vi "UHR-Fleezers Control (host) - 12.0_test_fpga_connection.vi"() -> ()   [LabVIEW 2014] (continued)
    }
    n2827 = feedback-in #12(w3586) -> ()
    n2828 = feedback-in #13(w3587) -> ()
    n2829 = Square Root(x=w3683) -> (sqrt(x)=w3682:dbl)
    n2830 = Or(x=w3868, y=w3864) -> (x .or. y?=w3865:bool)
    n2831 = Equal?(x="Tab Control 6", y=T41."High Res Display") -> (x = y?=w3800:bool)
    n2832 = Multiply(x="APD Disp. Scale", y=w3762) -> (x*y=w3771:waveform(dbl)[])
    n2833 = Multiply(x=10.0, y=w3682) -> (x*y=→"Trap 1 Position RMS (A)":dbl)
    n2834 = Multiply(x="APD Disp. Downsample", y=w3769) -> (x*y=w3767:dbl)
    n2835 = Divide(x=w3771, y=w3767) -> (x/y=w3741:waveform(dbl)[])
    n2836 = case "For displaying the high resolution display (no downsampling)" shown="True" w3800 {
      tunnel: w3766 -> [_ w4168]
      frame False {
      }
      frame True {
        n2837 = Index Array(array=w4168, index="High Res. Display") -> (element=w4169:waveform(dbl))
        n2838 = call <vilib>:"Std Deviation and Variance.vi"("X"=w4169) -> ("mean"=w4176:dbl, "standard deviation"=w4181:dbl)  [unwired: 1 in, 1 out]
        "Mean Intensity" <- w4176
        "Sigma" <- w4181
        n2839 = Subtract(x=w4169, y=w4176) -> (x-y=w4175:waveform(dbl))
        n2840 = Select(t=w4175, s="Subtract mean", f=w4169) -> (s? t:f=→"1 Channel":waveform(dbl))
        n2841 = Divide(x=w4181, y=w4176) -> (x/y=→"Sigma/Mean":dbl)
        n2842 = feedback #15(1) -> (w4170:i32)
        n2843 = Greater Or Equal?(x=w4170, y="Slow mean N ave.") -> (x >= y?=w4183:bool)
        n2844 = Increment(x=w4170) -> (x+1=w4185:i32)
        n2845 = Select(t=1, s=w4183, f=w4185) -> (s? t:f=w4172:i32)
        n2846 = feedback-in #15(w4172) -> ()
        n2847 = feedback #16() -> (w4173:waveform(dbl))  [unwired: 1 out]
        n2848 = case shown="Default" w4170 {
          tunnel: [w4188 w4191] -> w4174
          tunnel: w4173 -> [w4190 _]
          tunnel: w4169 -> [w4189 w4191]
          frame Default {
            n2849 = call-poly <vilib>:"Append Waveforms.vi"("waveform B"=w4189, "waveform A"=w4190) -> ("waveform out"=w4188:waveform(dbl))  [unwired: 1 in, 8 out]
          }
          frame 1 {
          }
        }
        n2850 = feedback-in #16(w4174) -> ()
        n2851 = case shown="True" w4183 {
          tunnel: w4174 -> [_ w4187]
          frame False {
          }
          frame True {
            n2852 = call-poly <vilib>:"Mean.vi"("X"=w4187) -> ("mean"=→"Slow mean":dbl)  [unwired: 1 out]
          }
        }
      }
    }
    n2853 = Index Array(array=w3741, index=0) -> (element=w3750:waveform(dbl))
    n2854 = Index Array(array=w3741, index=1) -> (element=w3748:waveform(dbl))
    n2855 = case "For computing FFTs for display" shown="True" "Compute FFT" {
      tunnel: w3766 -> [_ w4882]
      frame False {
      }
      frame True {
        n2856 = Build Array("FFT 1 Choice 1", "FFT 1 Choice 2", "FFT 2 Choice 1", "FFT 2 Choice 2") -> (w4875:u16[])
        n2857 = Array Size(array=w4882) -> (size(s)=w4881:i32)
        n2858 = feedback-in #17(w4875) -> ()
        n2859 = feedback #17(u16[] [100, 100, 100, 100]) -> (w4876:u16[])
        n2860 = feedback-in #18("# Spectra to Ave.") -> ()
        n2861 = feedback #18("# Spectra to Ave.") -> (w4873:dbl)
        n2862 = Not Equal?(x="# Spectra to Ave.", y=w4873) -> (x != y?=w4872:bool)
        n2863 = Not Equal?(x=w4875, y=w4876) -> (x != y?=w4874:bool)
        n2864 = feedback #19(1.0) -> (w4859:dbl)
        n2865 = Compound Arithmetic op=OR("Reset FFT", w4874, w4872) -> (w4857:bool)
        n2866 = Select(t=1.0, s=w4857, f=w4859) -> (s? t:f=w4861:dbl)
        n2867 = Greater?(x=w4861, y="# Spectra to Ave.") -> (0:w4880:bool)
        n2868 = Increment(x=w4861) -> (x+1=w4860:dbl)
        n2869 = feedback-in #19(w4860) -> ()
        n2870 = local read "DMA Update Period (s)"() -> (w4855:dbl)
        n2871 = Multiply(x="# Spectra to Ave.", y=w4855) -> (x*y=→"Ave. Time (s)":dbl)
        n2872 = Build Array(cluster{"f0":dbl, "df":dbl, "magnitude":dbl[]} {"f0"=0.0, "df"=0.0, "magnitude"=[]} ("PSD")) -> (w4864:cluster{"f0":dbl, "df":dbl, "magnitude":dbl[]}[])
        n2873 = Build Array(w4864, w4864, w4864, w4864) -> (w4866:T52)
        n2874 = feedback #20(w4866) -> (w4871:T52)
        n2875 = for {
          N: 4 -> [_]
          tunnel: w4875 -> [w4904] mode=indexing
          tunnel: w4882 -> [w4905]
          tunnel: w4881 -> [w4907]
          tunnel: w4857 -> [w4900]
          tunnel: w4880 -> [w4899]
          tunnel: "# Spectra to Ave." -> [w4898]
          tunnel: [w4897] -> w4870 mode=indexing
          tunnel: w4871 -> [w4902] mode=indexing
          tunnel: [w4901] -> w4858 mode=indexing
          tunnel: w4861 -> [w4896]
          n2876 = Less?(x=w4904, y=w4907) -> (x < y?=w4906:bool)
          n2877 = Index Array(array=w4905, index=w4904) -> (element=w4903:waveform(dbl))
          n2878 = case shown="True" w4906 {
            tunnel: w4903 -> [_ w4924]
            tunnel: w4902 -> [w4909 w4922]
            tunnel: [w4909 w4910] -> w4901
            tunnel: w4900 -> [_ w4921]
            tunnel: w4899 -> [_ w4914]
            tunnel: w4898 -> [_ w4913]
            tunnel: [cluster{"f0":dbl, "df":dbl, "magnitude":dbl[]} {"f0"=0.0, "df"=0.0, "magnitude"=[]} ("PSD") w4915] -> w4897
            tunnel: w4896 -> [_ w4912]
            frame False {
            }
            frame True {
              n2879 = call <vilib>:"Std Deviation and Variance.vi"("X"=w4924) -> ("mean"=w4925:dbl)  [unwired: 1 in, 2 out]
              n2880 = Subtract(x=w4924, y=w4925) -> (x-y=w4923:waveform(dbl))
              n2881 = xnode "Spectral Measurements"("Signals"=w4923) -> ("PSD"=w4917:cluster{"f0":dbl, "df":dbl, "magnitude":dbl[]})  [unwired: 1 in, 1 out]
              n2882 = case shown="False" w4921 {
                tunnel: w4922 -> [w4934 _]
                tunnel: [w4930 w4939] -> w4910
                tunnel: w4917 -> [w4933 w4940]
                tunnel: w4914 -> [w4932 _]
                frame False {
                  n2883 = Build Array (concatenate)(w4934, w4933) -> (w4931:cluster{"f0":dbl, "df":dbl, "magnitude":dbl[]}[])
                  n2884 = case shown="True" w4932 {
                    tunnel: w4931 -> [w4935 w4938]
                    tunnel: [w4935 w4936] -> w4930
                    frame False {
                    }
                    frame True {
                      n2885 = Delete From Array(array=w4938, index=0) -> (array with subset deleted=w4936:cluster{"f0":dbl, "df":dbl, "magnitude":dbl[]}[])  [unwired: 1 in, 1 out]
                    }
                  }
                }
                frame True {
                  n2886 = Build Array(w4940) -> (w4939:cluster{"f0":dbl, "df":dbl, "magnitude":dbl[]}[])
                }
              }
              n2887 = for {
                tunnel: w4910 -> [w4929] mode=indexing
                tunnel: [w4928] -> w4920 mode=indexing
                workers-P: _ -> [_]
                n2888 = Unbundle By Name(w4929) -> ("magnitude"=w4928:dbl[])
              }
              n2889 = Transpose 2D Array(2D array=w4920) -> (transposed array=w4919:dbl[][])
              n2890 = for {
                tunnel: w4919 -> [w4927] mode=indexing
                tunnel: [w4926] -> w4918 mode=indexing
                workers-P: _ -> [_]
                n2891 = Add Array Elements(numeric array=w4927) -> (sum=w4926:dbl)
              }
              n2892 = Select(t=w4913, s=w4914, f=w4912) -> (s? t:f=w4911:dbl)
              n2893 = Divide(x=w4918, y=w4911) -> (x/y=w4916:dbl[])
              n2894 = Bundle By Name(cluster=w4917, "magnitude"=w4916) -> (w4915:cluster{"f0":dbl, "df":dbl, "magnitude":dbl[]})
            }
          }
        }
        n2895 = case shown="True" w4857 {
          tunnel: w4858 -> [w4889 w4895]
          tunnel: [w4889 w4890] -> w4856
          frame False {
          }
          frame True {
            n2896 = Array Subset(array=w4895, index (row)=0 ("index"), length (row)=4 ("length"), index (col)=0 ("index"), length (col)=1 ("length")) -> (w4890:T52)
          }
        }
        n2897 = feedback-in #20(w4856) -> ()
        n2898 = Split 1D Array(array=w4870, index=2) -> (first subarray=→"FFT 1":cluster{"f0":dbl, "df":dbl, "magnitude":dbl[]}[], second subarray=→"FFT 2":cluster{"f0":dbl, "df":dbl, "magnitude":dbl[]}[])
      }
    }
    n2899 = case "For plotting results of scanning MCL" shown="True" w3865 {
      tunnel: w3864 -> [_ w4310]
      tunnel: w3794 -> [_ w4406]
      tunnel: w3873 -> [_ _]
      tunnel: w3766 -> [_ w4380]
      tunnel: w3743 -> [_ w4311]
      tunnel: w3742 -> [_ w4284]
      frame False {
      }
      frame True {
        w4291 = u32 0 items=["Horizontal", "Vertical", "Central", "1st Diagonal", "2nd Diagonal"] ("Type of Symmetry")
        w4319 = u32 0 items=["Horizontal", "Vertical", "Central", "1st Diagonal", "2nd Diagonal"] ("Type of Symmetry")
        w4322 = u32 0 items=["Horizontal", "Vertical", "Central", "1st Diagonal", "2nd Diagonal"] ("Type of Symmetry")
        w4351 = u32 0 items=["Horizontal", "Vertical", "Central", "1st Diagonal", "2nd Diagonal"] ("Type of Symmetry")
        n2900 = Index Array(array=w4380, index=10) -> (element=w4386:waveform(dbl))
        n2901 = Index Array(array=w4380, index=11) -> (element=w4383:waveform(dbl))
        n2902 = local read "Cycles/step (MCL)"() -> (w4336:u64)
        n2903 = Index Array(array=w4380, index="Channel") -> (element=w4382:waveform(dbl))
        n2904 = Unbundle(w4284) -> ("New Image"=w4283:T2, "New Image"=w4282:T2, "New Image"=w4281:T2, "New Image"=w4280:T2)
        n2905 = Unbundle By Name(w4386) -> ("Y"=w4338:dbl[])
        n2906 = Unbundle By Name(w4383) -> ("Y"=w4340:dbl[])
        n2907 = Unbundle By Name(w4382) -> ("Y"=w4345:dbl[])
        n2908 = call "downsample 1D array - double.vi"("Ave N"=w4336, "Array In"=w4338) -> ("Array Out"=w4337:dbl[])  [unwired: 1 out]
        n2909 = call "downsample 1D array - double.vi"("Ave N"=w4336, "Array In"=w4340) -> ("Array Out"=w4339:dbl[])  [unwired: 1 out]
        n2910 = call "downsample 1D array - double.vi"("Ave N"=w4336, "Array In"=w4345) -> ("Array Out"=w4344:dbl[])  [unwired: 1 out]
        n2911 = feedback #21(w4406) -> (w4407:dbl[])
        n2912 = Build Array (concatenate)(w4407, w4406) -> (w4388:dbl[])
        n2913 = feedback #22(w4311) -> (w4313:dbl[])
        n2914 = Build Array (concatenate)(w4313, w4311) -> (w4312:dbl[])
        n2915 = local read "Scan steps (MCL)"() -> (w4293:u64)
        n2916 = Select(t=w4406, s=w4310, f=w4388) -> (s? t:f=w4392:dbl[])
        n2917 = feedback-in #21(w4392) -> ()
        n2918 = Select(t=w4311, s=w4310, f=w4312) -> (s? t:f=w4294:dbl[])
        n2919 = feedback-in #22(w4294) -> ()
        n2920 = local read "Scan lines (y)"() -> (w4279:u64)
        n2921 = local read "N APD Samp/step"() -> (w4295:dbl)
        n2922 = feedback #23(w4337) -> (w4394:dbl[])
        n2923 = Build Array (concatenate)(w4394, w4337) -> (w4385:dbl[])
        n2924 = feedback #24(w4344) -> (w4404:dbl[])
        n2925 = Build Array (concatenate)(w4404, w4344) -> (w4403:dbl[])
        n2926 = feedback #25(w4339) -> (w4396:dbl[])
        n2927 = Build Array (concatenate)(w4396, w4339) -> (w4397:dbl[])
        n2928 = Select(t=w4337, s=w4310, f=w4385) -> (s? t:f=w4341:dbl[])
        n2929 = feedback-in #23(w4341) -> ()
        n2930 = Select(t=w4344, s=w4310, f=w4403) -> (s? t:f=w4343:dbl[])
        n2931 = feedback-in #24(w4343) -> ()
        n2932 = Select(t=w4339, s=w4310, f=w4397) -> (s? t:f=w4342:dbl[])
        n2933 = feedback-in #25(w4342) -> ()
        n2934 = Multiply(x=w4293, y=u64 2) -> (x*y=w4278:u64)
        n2935 = call "integrate 1D array interval - double.vi"("Ave N"=w4295, "Array In"=w4294) -> ("Array Out"=w4306:dbl[])  [unwired: 1 out]
        n2936 = call "integrate 1D array interval - double.vi"("Ave N"=w4295, "Array In"=w4392) -> ("Array Out"=w4391:dbl[])  [unwired: 1 out]
        n2937 = Array Size(array=w4306) -> (size(s)=w4307:i32)
        n2938 = Array Size(array=w4391) -> (size(s)=w4393:i32)
        n2939 = Multiply(x=w4279, y=w4278) -> (x*y=w4309:u64)
        n2940 = Multiply(x=w4279, y=w4278) -> (x*y=w4401:u64)
        n2941 = call-poly <vilib>:"Mean.vi"("X"=w4341) -> ("mean"=w4325:dbl)  [unwired: 1 out]
        n2942 = Subtract(x=w4309, y=w4307) -> (x-y=w4300:u64)
        n2943 = call-poly <vilib>:"Mean.vi"("X"=w4343) -> ("mean"=w4330:dbl)  [unwired: 1 out]
        n2944 = call-poly <vilib>:"Mean.vi"("X"=w4342) -> ("mean"=w4328:dbl)  [unwired: 1 out]
        n2945 = call-poly <vilib>:"Mean.vi"("X"=w4306) -> ("mean"=w4297:dbl)  [unwired: 1 out]
        n2946 = Subtract(x=w4401, y=w4393) -> (x-y=w4335:u64)
        n2947 = call-poly <vilib>:"Mean.vi"("X"=w4391) -> ("mean"=w4332:dbl)  [unwired: 1 out]
        n2948 = Initialize Array(1.0 ("element"), w4300) -> (w4296:dbl[])
        n2949 = Initialize Array(1.0 ("element"), w4335) -> (w4326:dbl[])
        n2950 = Multiply(x=w4296, y=w4297) -> (x*y=w4298:dbl[])
        n2951 = Multiply(x=w4326, y=w4328) -> (x*y=w4329:dbl[])
        n2952 = Multiply(x=w4326, y=w4330) -> (x*y=w4331:dbl[])
        n2953 = Multiply(x=w4326, y=w4325) -> (x*y=w4327:dbl[])
        n2954 = Multiply(x=w4326, y=w4332) -> (x*y=w4333:dbl[])
        n2955 = Build Array (concatenate)(w4341, w4327) -> (w4395:dbl[])
        n2956 = Build Array (concatenate)(w4343, w4331) -> (w4399:dbl[])
        n2957 = Build Array (concatenate)(w4342, w4329) -> (w4398:dbl[])
        n2958 = Build Array (concatenate)(w4306, w4298) -> (w4308:dbl[])
        n2959 = Build Array (concatenate)(w4391, w4333) -> (w4400:dbl[])
        n2960 = Reshape Array(w4395, w4279, w4278) -> (w4361:dbl[][])
        n2961 = Reshape Array(w4308, w4279, w4278) -> (w4304:dbl[][])
        n2962 = Reshape Array(w4399, w4279, w4278) -> (w4353:dbl[][])
        n2963 = Reshape Array(w4398, w4279, w4278) -> (w4368:dbl[][])
        n2964 = Reshape Array(w4400, w4279, w4278) -> (w4378:dbl[][])
        n2965 = Array Subset(array=w4368, index (col)=0 ("index"), length (col)=w4293) -> (w4373:dbl[][])  [unwired: 2 in]
        n2966 = Array Subset(array=w4368, index (col)=w4293) -> (w4371:dbl[][])  [unwired: 3 in]
        n2967 = Array Subset(array=w4353, index (col)=0 ("index"), length (col)=w4293) -> (w4359:dbl[][])  [unwired: 2 in]
        n2968 = Array Subset(array=w4353, index (col)=w4293) -> (w4357:dbl[][])  [unwired: 3 in]
        n2969 = Array Subset(array=w4304, index (col)=0 ("index"), length (col)=w4293) -> (w4303:dbl[][])  [unwired: 2 in]
        n2970 = Array Subset(array=w4304, index (col)=w4293) -> (w4301:dbl[][])  [unwired: 3 in]
        n2971 = Array Subset(array=w4378, index (col)=0 ("index"), length (col)=w4293) -> (w4377:dbl[][])  [unwired: 2 in]
        n2972 = Array Subset(array=w4378, index (col)=w4293) -> (w4375:dbl[][])  [unwired: 3 in]
        n2973 = Array Subset(array=w4361, index (col)=0 ("index"), length (col)=w4293) -> (w4366:dbl[][])  [unwired: 2 in]
        n2974 = Array Subset(array=w4361, index (col)=w4293) -> (w4364:dbl[][])  [unwired: 3 in]
        n2975 = for {
          tunnel: w4373 -> [w4415] mode=indexing
          tunnel: [w4414] -> w4372 mode=indexing
          workers-P: _ -> [_]
          n2976 = Reverse 1D Array(array=w4415) -> (reversed array=w4414:dbl[])
        }
        n2977 = for {
          tunnel: w4359 -> [w4411] mode=indexing
          tunnel: [w4410] -> w4358 mode=indexing
          workers-P: _ -> [_]
          n2978 = Reverse 1D Array(array=w4411) -> (reversed array=w4410:dbl[])
        }
        n2979 = for {
          tunnel: w4303 -> [w4409] mode=indexing
          tunnel: [w4408] -> w4302 mode=indexing
          workers-P: _ -> [_]
          n2980 = Reverse 1D Array(array=w4409) -> (reversed array=w4408:dbl[])
        }
        n2981 = for {
          tunnel: w4377 -> [w4417] mode=indexing
          tunnel: [w4416] -> w4376 mode=indexing
          workers-P: _ -> [_]
          n2982 = Reverse 1D Array(array=w4417) -> (reversed array=w4416:dbl[])
        }
        n2983 = for {
          tunnel: w4366 -> [w4413] mode=indexing
          tunnel: [w4412] -> w4365 mode=indexing
          workers-P: _ -> [_]
          n2984 = Reverse 1D Array(array=w4413) -> (reversed array=w4412:dbl[])
        }
        n2985 = Index Array(array=w4378, index (row)=0) -> (element=→"Waveform Graph":dbl[])  [unwired: 1 in]
        n2986 = Add(x=w4372, y=w4371) -> (x+y=w4370:dbl[][])
        n2987 = Add(x=w4358, y=w4357) -> (x+y=w4356:dbl[][])
        n2988 = Add(x=w4302, y=w4301) -> (x+y=w4286:dbl[][])
        n2989 = Add(x=w4376, y=w4375) -> (x+y=w4350:dbl[][])
        n2990 = Add(x=w4365, y=w4364) -> (x+y=w4363:dbl[][])
        n2991 = Divide(x=w4356, y=2) -> (x/y=w4354:dbl[][])
        n2992 = Divide(x=w4370, y=2) -> (x/y=w4315:dbl[][])
        n2993 = Divide(x=w4363, y=2) -> (x/y=w4317:dbl[][])
        n2994 = To Single Precision Float(number=w4350) -> (single precision float=w4349:sgl[][])
        n2995 = Transpose 2D Array(2D array=w4354) -> (transposed array=→"Data map":dbl[][])
        n2996 = To Single Precision Float(number=w4286) -> (single precision float=w4290:sgl[][])
        n2997 = To Single Precision Float(number=w4315) -> (single precision float=w4321:sgl[][])
        n2998 = To Single Precision Float(number=w4317) -> (single precision float=w4318:sgl[][])
        n2999 = call "IMAQ ArrayToImage"("Image Pixels (Float)"=w4349, "Image"=w4283) -> ("Image Out"=w4352:T2)  [unwired: 8 in, 1 out]
        n3000 = call "IMAQ ArrayToImage"("Image Pixels (Float)"=w4290, "Image"=w4282) -> ("Image Out"=w4292:T2)  [unwired: 8 in, 1 out]
        n3001 = call "IMAQ ArrayToImage"("Image Pixels (Float)"=w4321, "Image"=w4281) -> ("Image Out"=w4323:T2)  [unwired: 8 in, 1 out]
        n3002 = call "IMAQ ArrayToImage"("Image Pixels (Float)"=w4318, "Image"=w4280) -> ("Image Out"=w4320:T2)  [unwired: 8 in, 1 out]
        n3003 = call "IMAQ Symmetry"("Type of Symmetry"=w4351, "Image Src"=w4352) -> ("Image Dst Out"=w4347:T2)  [unwired: 3 in, 1 out]
        n3004 = call "IMAQ Symmetry"("Type of Symmetry"=w4291, "Image Src"=w4292) -> ("Image Dst Out"=w4288:T2)  [unwired: 3 in, 1 out]
        n3005 = call "IMAQ Symmetry"("Type of Symmetry"=w4322, "Image Src"=w4323) -> ("Image Dst Out"=→"Detection Laser X":T2)  [unwired: 3 in, 1 out]
        n3006 = call "IMAQ Symmetry"("Type of Symmetry"=w4319, "Image Src"=w4320) -> ("Image Dst Out"=→"Detection Laser Y":T2)  [unwired: 3 in, 1 out]
        n3007 = call "IMAQ Set Simple Calibration"("Calibration Axis Info"=T42 {"Origin Pixel"={"X"=0.0, "Y"=0.0}, "Angle Relative to Horizontal (deg)"=0.0, "Axis Reference"=0}, "Grid Descriptor"=T43 {"X Step"=0.3, "Y Step"=0.3, "Unit"=enum."Undefined"}, "Image"=w4347) -> ("Calibrated Image"=→"APD 1":T2)  [unwired: 7 in, 1 out]
        n3008 = call "IMAQ Set Simple Calibration"("Calibration Axis Info"=T42 {"Origin Pixel"={"X"=0.0, "Y"=0.0}, "Angle Relative to Horizontal (deg)"=0.0, "Axis Reference"=0}, "Grid Descriptor"=T43 {"X Step"=0.3, "Y Step"=0.3, "Unit"=enum."Undefined"}, "Image"=w4288) -> ("Calibrated Image"=→"APD 2":T2)  [unwired: 7 in, 1 out]
      }
    }
    n3009 = Subtract(x=w3748, y="APD 2 Offset") -> (x-y=w3745:waveform(dbl))
    n3010 = Subtract(x=w3750, y="APD 1 Offset") -> (x-y=w3746:waveform(dbl))
    n3011 = Index Array(array=w3764, index=3) -> (element=w3818:waveform(dbl))
    n3012 = Index Array(array=w3764, index=6) -> (element=w3815:waveform(dbl))
    n3013 = Build Array(w3746, w3745) -> (→"APD Chart":waveform(dbl)[])
    n3014 = Array Size(array=w3586) -> (size(s)=w3854:i32)
    n3015 = call <vilib>:"Std Deviation and Variance.vi"("X"=w3587) -> ("standard deviation"=w3757:dbl)  [unwired: 1 in, 2 out]
    n3016 = Add Array Elements(numeric array=w3587) -> (sum=w3759:u32)
    n3017 = Add Array Elements(numeric array=w3586) -> (sum=w3863:u32)
    n3018 = call <vilib>:"Std Deviation and Variance.vi"("X"=w3586) -> ("standard deviation"=w3809:dbl)  [unwired: 1 in, 2 out]
    n3019 = Divide(x="T1 offset_x (mV)", y=1000.0) -> (x/y=w3819:dbl)
    n3020 = Divide(x=w3757, y=w3756) -> (x/y=w3753:dbl)
    "Rate sigma (Hz) 2" <- w3753
    n3021 = Multiply(x=w3756, y=w3854) -> (x*y=w3758:dbl)
    "Int. Time (s)" <- w3758
    n3022 = Divide(x=w3759, y=w3758) -> (x/y=w3754:dbl)
    "APD 2 Rate (Hz)" <- w3754
    n3023 = Divide(x=w3863, y=w3758) -> (x/y=w3807:dbl)
    "APD 1 Rate (Hz)" <- w3807
    n3024 = Divide(x=w3809, y=w3756) -> (x/y=w3808:dbl)
    "Rate sigma (Hz)" <- w3808
    n3025 = Divide(x=w3753, y=w3754) -> (x/y=→"Sigma/Mean 2":dbl)
    n3026 = Divide(x=w3808, y=w3807) -> (x/y=→"s/Mean":dbl)
    n3027 = feedback-in #26("Calibration") -> ()
    n3028 = feedback #26(u16 1 ("Calibration")) -> (w3837:u16)
    n3029 = Divide(x="T2 offset_x (mV)", y=1000.0) -> (x/y=w3817:dbl)
    n3030 = case shown="0, Default" "Calibration" {
      tunnel: "T1 a_x (nm/V)" -> [_ w4246 w4267]
      tunnel: "T1 k_x (pN/nm)" -> [_ _ w4257]
      tunnel: "T2 a_x (nm/V)" -> [_ w4245 w4265]
      tunnel: "T2 k_x (pN/nm)" -> [_ _ w4258]
      tunnel: w3818 -> [w4228 w4243 w4263]
      tunnel: w3815 -> [w4227 w4241 w4261]
      tunnel: [w4228 w4240 w4260] -> w3846
      tunnel: [w4227 w4239 w4259] -> w3845
      tunnel: ["T1 X (V)" ("Label.Text") "T1 X (nm)" ("Label.Text") "T1 X (pN)" ("Label.Text")] -> w3834
      tunnel: ["T2 X (V)" ("Label.Text") "T2 X (nm)" ("Label.Text") "T2 X (pN)" ("Label.Text")] -> w3833
      tunnel: ["Position (V)" ("Label.Text") "Position (nm)" ("Label.Text") "Force (pN)" ("Label.Text")] -> w3835
      tunnel: w3817 -> [_ w4231 w4250]
      tunnel: w3819 -> [_ w4234 w4252]
      tunnel: ["Mean (V)" ("Label.Text") "Mean (nm)" ("Label.Text") "Mean (pN)" ("Label.Text")] -> w3830
      tunnel: ["Difference (V)" ("Label.Text") "Difference (nm)" ("Label.Text") "Difference (pN)" ("Label.Text")] -> w3772
      frame 0, Default {
      }
      frame 1 {
        n3031 = Unbundle By Name(w4243) -> ("Y"=w4247:dbl[])
        n3032 = Unbundle By Name(w4241) -> ("Y"=w4232:dbl[])
        n3033 = Subtract(x=w4247, y=w4234) -> (x-y=w4235:dbl[])
        n3034 = Subtract(x=w4232, y=w4231) -> (x-y=w4233:dbl[])
        n3035 = Multiply(x=w4233, y=w4245) -> (x*y=w4242:dbl[])
        n3036 = Multiply(x=w4246, y=w4235) -> (x*y=w4244:dbl[])
        n3037 = Bundle By Name(cluster=w4241, "Y"=w4242) -> (w4239:waveform(dbl))
        n3038 = Bundle By Name(cluster=w4243, "Y"=w4244) -> (w4240:waveform(dbl))
      }
      frame 2 {
        n3039 = Unbundle By Name(w4263) -> ("Y"=w4268:dbl[])
        n3040 = Unbundle By Name(w4261) -> ("Y"=w4266:dbl[])
        n3041 = Subtract(x=w4266, y=w4250) -> (x-y=w4251:dbl[])
        n3042 = Subtract(x=w4268, y=w4252) -> (x-y=w4253:dbl[])
        n3043 = Compound Arithmetic op=MULTIPLY(w4251, w4265, w4258) -> (w4262:dbl[])
        n3044 = Compound Arithmetic op=MULTIPLY(w4257, w4267, w4253) -> (w4264:dbl[])
        n3045 = Bundle By Name(cluster=w4261, "Y"=w4262) -> (w4259:waveform(dbl))
        n3046 = Bundle By Name(cluster=w4263, "Y"=w4264) -> (w4260:waveform(dbl))
      }
    }
    n3047 = Not Equal?(x=w3837, y="Calibration") -> (x != y?=w3798:bool)
    n3048 = case shown="True" w3798 {
      tunnel: w3835 -> [_ w4221]
      tunnel: w3834 -> [_ w4220]
      tunnel: w3833 -> [_ w4219]
      tunnel: w3830 -> [_ w4218]
      tunnel: w3772 -> [_ w4217]
      frame False {
      }
      frame True {
        n3049 = property on="Force" class="WFChart (strict)"("YScale.NameLbl.Text"=w4221) -> ()  [unwired: 2 in, 2 out]
        n3050 = property on="T2 X" class="DigNum (strict)"("Caption.Text"=w4219) -> ()  [unwired: 2 in, 2 out]
        n3051 = property on="T1 X" class="DigNum (strict)"("Caption.Text"=w4220) -> ()  [unwired: 2 in, 2 out]
        n3052 = property on="Mean" class="DigNum (strict)"("Caption.Text"=w4218) -> ()  [unwired: 2 in, 2 out]
        n3053 = property on="Difference" class="DigNum (strict)"("Caption.Text"=w4217) -> ()  [unwired: 2 in, 2 out]
      }
    }
    n3054 = Unbundle By Name(w3818) -> ("Y"=w3821:dbl[])
    n3055 = Unbundle By Name(w3815) -> ("Y"=w3824:dbl[])
    n3056 = Subtract(x=w3821, y=w3819) -> (x-y=w3822:dbl[])
    n3057 = Subtract(x=w3824, y=w3817) -> (x-y=w3823:dbl[])
    n3058 = Multiply(x=w3823, y="T2 a_x (nm/V)") -> (x*y=w3625:dbl[])
    n3059 = Multiply(x="T1 a_x (nm/V)", y=w3822) -> (x*y=w3626:dbl[])
    n3060 = Not(x="Trap Trig. Fl.") -> (.not. x?=w3662:bool)
    n3061 = Multiply(x=w3845, y=-1.0) -> (x*y=w3826:waveform(dbl))
    n3062 = Subtract(x=w3626, y=w3625) -> (x-y=w3814:dbl[])
    n3063 = Unbundle By Name(w3845) -> ("Y"=w3788:dbl[])
    n3064 = Unbundle By Name(w3846) -> ("Y"=w3627:dbl[])
    n3065 = Negate(x=w3814) -> (-x=w3623:dbl[])
    n3066 = Build Array(w3846, w3826) -> (→"Force":waveform(dbl)[])
    n3067 = Subtract(x=w3623, y="Offset (nm)") -> (x-y=w3786:dbl[])
    n3068 = case shown="True" "Read Lateness and Rel Phase" {
      tunnel: w3643 -> [w4192 w4216]
      tunnel: w3642 -> [w4193 w4215]
      tunnel: [w4192 w4214] -> w3812
      tunnel: [w4193 w4213] -> w3811
      frame False {
      }
      frame True {
        n3069 = xnode "Read/Write Control"("FPGA VI Reference In"=w4216, "error in"=w4215) -> ("FPGA VI Reference Out"=w4214:T22, "error out"=w4213:errorcluster, "GI Relative phase"=→"GI relative phase":i16, "Relative phase"=→"Relative phase (AI1)":i16, "AI Late Counter"=→"Late Counter (AI1)":u8, "GI Late Counter"=→"GI Late Counter":u8, "MCL Late Counter"=→"MCL Late Counter":u8, "MCL Relative Phase"=→"Relative Phase (MCL)":i16, "APD Acq Relative Phase"=→"APD Acq Relative Phase":i16, "APD 1 Gate Relative Phase"=→"APD 1 Gate Relative Phase":i16, "APD 2 Gate Relative Phase"=→"APD 2 Gate Relative Phase":i16, "APD Acq Late Counter"=→"APD Acq Late Counter":u8, "APD 1 Gate Late Counter"=→"APD 1 Gate Late Counter":u8, "APD 2 Gate Late Counter"=→"APD 2 Gate Late Counter":u8, "Green FB Relative Phase"=→"Relative phase (Green FB)":i16, "GI Relative phase 2"=→"GI relative phase 2":i16, "GI Late Counter 2"=→"GI Late Counter 2":u8, "Trap Pos FIFO Timeout"=→"Trap Pos FIFO Timeout":u16, "Trap AI FIFO Timeout"=→"Trap AI FIFO Timeout":u16, "RI relative phase"=→"RI relative phase":i16, "RI late counter"=→"RI late counter":u8)
      }
    }
    n3070 = call-poly <vilib>:"Mean.vi"("X"=w3788) -> ("mean"=w3629:dbl)  [unwired: 1 out]
    "T2 X" <- w3629
    n3071 = Negate(x=w3788) -> (-x=w3789:dbl[])
    n3072 = call-poly <vilib>:"Mean.vi"("X"=w3627) -> ("mean"=w3630:dbl)  [unwired: 1 out]
    "T1 X" <- w3630
    n3073 = Negate(x=w3629) -> (-x=w3628:dbl)
    n3074 = Bundle By Name(cluster=w3818, "Y"=w3786) -> (w3763:waveform(dbl))
    "Bead Separation" <- w3763
    n3075 = Add(x=w3627, y=w3789) -> (x+y=w3790:dbl[])
    n3076 = Add(x=w3630, y=w3628) -> (x+y=w3832:dbl)
    n3077 = Subtract(x=w3630, y=w3628) -> (x-y=→"Difference":dbl)
    n3078 = Divide(x=w3790, y=2.0) -> (x/y=→"Vec Mean of T1 T2":dbl[])
    n3079 = Divide(x=w3832, y=2.0) -> (x/y=w3792:dbl)
    "Mean" <- w3792
    n3080 = feedback-in #27("Trap Trig. Fl.") -> ()
    n3081 = feedback #27("Trap Trig. Fl.") -> (w3660:bool)
    n3082 = And(x=w3662, y=w3660) -> (x .and. y?=w3661:bool)
    n3083 = case "If have just turned off triggering" shown="True" w3661 {
      tunnel: w3643 -> [_ w4022]
      tunnel: w3642 -> [_ w4021]
      frame False {
      }
      frame True {
        w4020 = FALSE ("FPGA Trap Trig")
        n3084 = xnode "Read/Write Control"("FPGA VI Reference In"=w4022, "error in"=w4021, "FPGA Trap Trig"=w4020) -> ("FPGA VI Reference Out"=w4019:T22, "error out"=w4018:errorcluster)
        n3085 = xnode "Read/Write Control"("FPGA VI Reference In"=w4019, "error in"=w4018, "TTrig?"=w4020) -> ()  [unwired: 2 out]
        n3086 = local write "Initializing"(FALSE ("Initializing")) -> ()
        n3087 = local write "Triggered"(FALSE ("Triggered")) -> ()
        n3088 = local write "Waiting"(FALSE ("Waiting")) -> ()
      }
    }
    n3089 = Not(x=w3660) -> (.not. x?=w3673:bool)
    n3090 = And(x="Trap Trig. Fl.", y=w3673) -> (x .and. y?=w3670:bool)
    n3091 = local read "Tether"() -> (w3793:bool)
    n3092 = Or(x=w3670, y="Reinitialize") -> (x .or. y?=w3656:bool)
    n3093 = feedback #28(w3666) -> (w3671:string)
    n3094 = Select(t=w3666, s=w3670, f=w3671) -> (s? t:f=w3665:string)
    n3095 = Select(t=w3666, s="Reinitialize", f=w3665) -> (s? t:f=w3664:string)
    n3096 = feedback #29(0) -> (w3668:i32)
    n3097 = feedback #30(w3786) -> (w3785:dbl[])
    n3098 = Build Array (concatenate)(w3786, w3785) -> (w3624:dbl[])
    n3099 = case "For determining if there is a tether still" shown="True" w3793 {
      tunnel: w3792 -> [_ w4146]
      frame False {
      }
      frame True {
        n3100 = Greater?(x="Lost Tether Alarm Threshold (pN)", y=w4146) -> (0:w4144:bool)
        n3101 = case shown="True" w4144 {
          frame False {
          }
          frame True {
            w4147 = TRUE
            w4151 = FALSE ("Multiple tether")
            w4152 = FALSE ("Value (Signaling)")
            n3102 = flat-sequence {
              frame #0 {
                # "stop only if saving"
                n3103 = local read "Saving..."() -> (w4164:bool)
                n3104 = And(x=w4164, y="TA Cancel Save?") -> (x .and. y?=w4163:bool)
                n3105 = local write "Stop Saving"(w4163) -> ()
              }
              frame #1 {
                n3106 = case shown="True" "TA Green Off?" {
                  frame False {
                  }
                  frame True {
                    w4167 = FALSE ("Fl. Triggered...")
                    n3107 = local write "Fl. Triggered..."(w4167) -> ()
                    n3108 = property on="Green ON/Interlacing" class="Bool (strict)"("Val(Sgnl)"=w4167) -> ()  [unwired: 2 in, 2 out]
                  }
                }
              }
            }
            n3109 = local read "Time tether formed"() -> (w4158:timestamp)
            n3110 = Get Date/Time In Seconds() -> (seconds since 1Jan1904=w4159:timestamp)
            n3111 = Subtract(x=w4159, y=w4158) -> (x-y=w4157:dbl)
            n3112 = Number To Decimal String(number=w4157) -> (decimal integer string=w4154:string)  [unwired: 1 out]
            n3113 = local read "Messages"() -> (w4161:string)
            n3114 = call <vilib>:"Beep.vi"("use system alert? (T)"=FALSE, "duration (msec)"=u32 200, "frequency (Hz)"=u32 200) -> ()  [unwired: 9 out]
            n3115 = Concatenate Strings("Lost tether (" ("Message to add"), w4154, " s)." ("string")) -> (w4156:string)
            n3116 = local write "Tether"(FALSE ("Tether")) -> ()
            n3117 = call "Update messages.vi"("Message to add"=w4156, "Old message string"=w4161) -> ("New message string"=w4160:string)
            n3118 = local write "Messages"(w4160) -> ()
            n3119 = local write "Pause dwell"(w4152) -> ()
            n3120 = property on="Fl. Triggered..." class="Bool (strict)"("Val(Sgnl)"=w4152) -> ()  [unwired: 2 in, 2 out]
            n3121 = local write "Dip for Protein"(w4152) -> ()
            n3122 = property on="Trap Pos. FB ON" class="Bool (strict)"("Val(Sgnl)"=w4152) -> ()  [unwired: 2 in, 2 out]
            n3123 = property on="Trap Trig. Fl." class="Bool (strict)"("Val(Sgnl)"=w4152) -> ()  [unwired: 2 in, 2 out]
            n3124 = local write "Multiple tether"(w4151) -> ()
            n3125 = local write "Bad fit"(w4151) -> ()
            n3126 = local write "Hysteresis"(w4151) -> ()
            n3127 = local write "Good tether"(w4151) -> ()
            n3128 = local write "Save scans"(w4147) -> ()
            n3129 = local write "Restart DMA? (AOD)"(w4147) -> ()
          }
        }
      }
    }
    n3130 = case "For triggering actions based on the trap position (e.g., turning the excitation laser on if trap under feedback moves so far)" shown="True" "Trap Trig. Fl." {
      tunnel: w3651 -> [_ w4035]
      tunnel: w3664 -> [_ w4034]
      tunnel: ["" ("t") w4033] -> w3672
      tunnel: w3656 -> [_ w4032]
      tunnel: [0 ("t") w4031] -> w3669
      tunnel: w3668 -> [_ w4030]
      tunnel: w3643 -> [_ w4029]
      tunnel: w3642 -> [_ w4028]
      frame False {
      }
      frame True {
        n3131 = case shown="\"Wait for trigger\"" w4034 {
          tunnel: w4035 -> [w4052 _ _ w4100]
          tunnel: [w4049 w4081 "" ("t") w4103] -> w4033
          tunnel: w4032 -> [_ _ _ w4091]
          tunnel: [w4048 w4078 0 ("t") w4092] -> w4031
          tunnel: w4030 -> [_ w4080 _ w4098]
          tunnel: w4029 -> [w4037 w4075 _ w4094]
          tunnel: w4028 -> [w4036 w4074 _ w4093]
          frame "Wait for trigger" {
            n3132 = local read "Trap Trig. (FPGA)"() -> (w4040:bool)
            n3133 = Subtract(x=w4052, y="Mean T1 Position\nto compare (nm)") -> (x-y=w4045:dbl[])
            n3134 = call <vilib>:"Std Deviation and Variance.vi"("X"=w4045) -> ("mean"=→"mean":dbl, "standard deviation"=→"standard\ndeviation":dbl)  [unwired: 1 in, 1 out]
            n3135 = Array Max & Min(array=w4045) -> (max value=→"max value":dbl, min value=→"min value":dbl)  [unwired: 2 out]
            n3136 = Greater?(x=w4045, y="Threshold (nm)") -> (0:w4055:bool[])
            n3137 = case shown="True" w4040 {
              tunnel: w4037 -> [_ w4061]
              tunnel: w4036 -> [_ w4060]
              tunnel: [FALSE ("TTrig?") w4059] -> w4043
              frame False {
              }
              frame True {
                n3138 = xnode "Read/Write Control"("FPGA VI Reference In"=w4061, "error in"=w4060) -> ("TTrig?"=w4059:bool)  [unwired: 2 out]
              }
            }
            n3139 = Or Array Elements(Boolean array=w4055) -> (logical OR=w4042:bool)
            n3140 = Select(t=w4043, s=w4040, f=w4042) -> (s? t:f=w4041:bool)
            n3141 = Not(x=w4040) -> (.not. x?=w4039:bool)
            n3142 = And(x=w4041, y=w4039) -> (x .and. y?=w4038:bool)
            n3143 = Select(t="Triggered", s=w4041, f="Wait for trigger") -> (s? t:f=w4049:string)
            n3144 = case shown="True" w4041 {
              tunnel: [0 0] -> w4048
              tunnel: w4037 -> [_ w4066]
              tunnel: w4036 -> [_ w4065]
              frame False {
                "Waiting" <- TRUE ("Waiting")
              }
              frame True {
                n3145 = xnode "Read/Write Control"("FPGA VI Reference In"=w4066, "error in"=w4065, "TTrig?"=FALSE) -> ()  [unwired: 2 out]
                n3146 = local read "Messages"() -> (w4069:string)
                n3147 = call <vilib>:"Beep.vi"() -> ()  [unwired: 12 in]
                n3148 = call "Update messages.vi"("Message to add"="Unwinding trigger.", "Old message string"=w4069) -> ("New message string"=w4070:string)
                n3149 = local write "Messages"(w4070) -> ()
                n3150 = local write "Waiting"(FALSE ("Waiting")) -> ()
                "Triggered" <- TRUE ("Triggered")
              }
            }
            n3151 = case "Only need to turn on laser if host triggered" shown="True" w4038 {
              frame False {
              }
              frame True {
                n3152 = property on="Green ON/Interlacing" class="Bool (strict)"("Val(Sgnl)"=TRUE ("Value (Signaling)")) -> ()  [unwired: 2 in, 2 out]
              }
            }
          }
          frame "Triggered" {
            n3153 = local read "Trap Trig. (FPGA)"() -> (w4077:bool)
            n3154 = Increment(x=w4080) -> (x+1=w4078:i32)
            n3155 = Greater Or Equal?(x=w4078, y="Fl. ON time (n)") -> (x >= y?=w4076:bool)
            n3156 = Select(t="Wait for trigger", s=w4076, f="Triggered" ("t")) -> (s? t:f=w4081:string)
            n3157 = And(x=w4076, y=w4077) -> (x .and. y?=w4073:bool)
            n3158 = case shown="True" w4073 {
              tunnel: w4075 -> [_ w4085]
              tunnel: w4074 -> [_ w4084]
              frame False {
              }
              frame True {
                n3159 = xnode "Read/Write Control"("FPGA VI Reference In"=w4085, "error in"=w4084, "FPGA Trap Trig"=TRUE) -> ()  [unwired: 2 out]
              }
            }
            n3160 = case shown="True" w4076 {
              frame False {
              }
              frame True {
                w4087 = FALSE ("Value (Signaling)")
                n3161 = local write "Triggered"(w4087) -> ()
                n3162 = local write "Waiting"(TRUE ("Waiting")) -> ()
                n3163 = property on="Green ON/Interlacing" class="Bool (strict)"("Val(Sgnl)"=w4087) -> ()  [unwired: 2 in, 2 out]
              }
            }
          }
          frame "Do nothing" {
          }
          frame "Initialize", Default {
            n3164 = Increment(x=w4098) -> (x+1=w4102:i32)
            n3165 = Select(t=1, s=w4091, f=w4102) -> (s? t:f=w4092:i32)
            n3166 = feedback #31(w4100) -> (w4106:dbl[])
            n3167 = Build Array (concatenate)(w4100, w4106) -> (w4099:dbl[])
            n3168 = Greater Or Equal?(x=w4092, y="Wait to get offset (n)") -> (x >= y?=w4095:bool)
            n3169 = Select(t=w4100, s=w4091, f=w4099) -> (s? t:f=w4101:dbl[])
            n3170 = feedback-in #31(w4101) -> ()
            n3171 = call-poly <vilib>:"Mean.vi"("X"=w4101) -> ("mean"=w4096:dbl)  [unwired: 1 out]
            n3172 = local write "Mean T1 Position\nto compare (nm)"(w4096) -> ()
            n3173 = case shown="True" w4091 {
              tunnel: w4094 -> [_ w4112]
              tunnel: w4093 -> [_ w4111]
              frame False {
              }
              frame True {
                w4108 = FALSE ("FPGA Trap Trig")
                n3174 = xnode "Read/Write Control"("FPGA VI Reference In"=w4112, "error in"=w4111, "FPGA Trap Trig"=w4108) -> ("FPGA VI Reference Out"=w4110:T22, "error out"=w4109:errorcluster)
                n3175 = xnode "Read/Write Control"("FPGA VI Reference In"=w4110, "error in"=w4109, "TTrig?"=w4108) -> ()  [unwired: 2 out]
              }
            }
            n3176 = Select(t="Wait for trigger", s=w4095, f="Initialize") -> (s? t:f=w4103:string)
            n3177 = case shown="True" w4095 {
              tunnel: w4096 -> [_ w4115]
              tunnel: w4094 -> [_ w4124]
              tunnel: w4093 -> [_ w4123]
              frame False {
                n3178 = local write "Waiting"(FALSE ("Waiting")) -> ()
                "Initializing" <- TRUE ("Initializing")
              }
              frame True {
                n3179 = local read "Threshold (nm)"() -> (w4127:dbl)
                n3180 = local read "AOM X Cal (nm/MHz)"() -> (w4126:dbl)
                n3181 = Add(x=w4115, y=w4127) -> (x+y=w4128:dbl)
                n3182 = Divide(x=w4128, y=w4126) -> (x/y=w4125:dbl)
                n3183 = call "IR AOM freq to word.vi"("Frequency In (MHz)"=w4125) -> ("Frequency Word Out (double)"=w4122:dbl)
                n3184 = local write "Initializing"(FALSE ("Initializing")) -> ()
                n3185 = local write "Waiting"(TRUE ("Waiting")) -> ()
                n3186 = To Quad Integer(1:w4122) -> (0:w4121:i64)
                n3187 = xnode "Read/Write Control"("FPGA VI Reference In"=w4124, "error in"=w4123, "FPGA TTrig Thresh"=w4121) -> ("FPGA VI Reference Out"=w4118:T22, "error out"=w4117:errorcluster)
                n3188 = xnode "Read/Write Control"("FPGA VI Reference In"=w4118, "error in"=w4117, "FPGA Trap Trig"=TRUE) -> ()  [unwired: 2 out]
              }
            }
          }
        }
      }
    }
    n3189 = feedback-in #28(w3672) -> ()
    n3190 = feedback-in #29(w3669) -> ()
    n3191 = Split 1D Array(array=w3624, index=w3686) -> (first subarray=w3782:dbl[])  [unwired: 1 out]
    n3192 = feedback-in #30(w3782) -> ()
    n3193 = call-poly <vilib>:"Mean.vi"("X"=w3782) -> ("mean"=w3781:dbl)  [unwired: 1 out]
    "Bead Mean (nm)" <- w3781
    n3194 = Subtract(x=w3782, y=w3781) -> (x-y=w3780:dbl[])
    n3195 = Square(x=w3780) -> (x^2=w3779:dbl[])
    n3196 = call-poly <vilib>:"Mean.vi"("X"=w3779) -> ("mean"=w3778:dbl)  [unwired: 1 out]
    n3197 = Square Root(x=w3778) -> (sqrt(x)=w3777:dbl)
    n3198 = Multiply(x=10.0, y=w3777) -> (x*y=→"RMS (Å)":dbl)
    n3199 = xnode ("Read/Write Control")("FPGA VI Reference In"=w3812, "error in"=w3811) -> ("FPGA VI Reference Out"=w3654:T22, "error out"=w3653:errorcluster, "AI2 Y Sum Set 1"=w3907:i16, "AI2 Y Sum Set 2"=w3906:i16, "AI1 X Set 1"=w3714:fxp<+/-,16,1>, "AI1 X Set 2"=w3713:fxp<+/-,16,1>, "Trap Pos FB Int Signal"=→"Trap Pos FB Int Signal":fxp<+/-,24,9>, "Trap Pos FB Int-Norm Signal"=→"Trap Pos FB Int-Norm Signal":fxp<+/-,16,1>, "Trap Pos FB Action"=w3707:i64, "Scanning"=→"AOD Scanning":bool, "Scan I"=→"AOD Scan I":u64, "Scanning MCL"=w3909:bool, "Scan I (MCL)"=→"MCL Scan I":u64, "Green FB Sum"=w3849:i16, "Trap Pos FB Action"=w3641:i64, "Wiggling 1"=→"Wiggling T1":bool, "TTrig Fin Thresh"=w3637:i64, "Wiggling 2"=→"Wiggling T2":bool, "Red FB Sum"=w3604:i16)  [unwired: 2 out]
    "MCL Scanning" <- w3909
    "Trap Pos FB Action" <- w3707
    n3200 = local read "FB Trig Integrate"() -> (w3635:u32)
    n3201 = Divide(x=w3849, y=3276.7) -> (x/y=w3603:dbl)
    "Green laser intensity (V)" <- w3603
    n3202 = Divide(x=w3604, y=3276.7) -> (x/y=w3602:dbl)
    "Red laser intensity (V)" <- w3602
    n3203 = Divide(x=w3641, y=w3635) -> (x/y=w3634:dbl)
    "TTrig Sig (Int)" <- w3634
    n3204 = Divide(x=w3637, y=w3635) -> (x/y=w3632:dbl)
    "TTrig Fin Thresh (Int)" <- w3632
    n3205 = local read "AOM X Cal (nm/MHz)"() -> (w3640:dbl)
    n3206 = local read "AI2 (V)"() -> (w3908:cluster{"Set 1":dbl, "Set 2":dbl})
    n3207 = Bundle By Name(cluster=w3908, "Set 1"=w3907, "Set 2"=w3906) -> (w3904:cluster{"Set 1":dbl, "Set 2":dbl})
    n3208 = Divide(x=w3707, y=327.67) -> (x/y=w3619:dbl)
    n3209 = local read "Trap X (AI1)"() -> (w3727:T10)
    n3210 = Bundle(w3603, w3602) -> (→"Excitation laser intensities plot":cluster{dbl, dbl})  [unwired: 1 in]
    n3211 = call "IR AOM word double to freq.vi"("Frequency Word In (double)"=w3632) -> ("Frequency Out (MHz)"=w3631:dbl)
    n3212 = call "IR AOM word double to freq.vi"("Frequency Word In (double)"=w3634) -> ("Frequency Out (MHz)"=w3633:dbl)
    n3213 = Divide(x=w3904, y=3276.7) -> (x/y=w3903:cluster{"Set 1":dbl, "Set 2":dbl})
    n3214 = Multiply(x=w3633, y=w3640) -> (x*y=w3639:dbl)
    "TTrig Sig (nm)" <- w3639
    n3215 = Multiply(x=w3631, y=w3640) -> (x*y=w3638:dbl)
    "TTrig Fin Thresh (nm)" <- w3638
    n3216 = local write "AI2 (V)"(w3903) -> ()
    n3217 = local read "Trap Pos. FB Range"() -> (w3618:T12)
    n3218 = Bundle(cluster=w3727, "Trap 1"=w3714, "Trap 2"=w3713) -> (→"Trap X (AI1)":T10)
    n3219 = Bundle(w3639, w3638) -> (→"TTrig":cluster{dbl, dbl})  [unwired: 1 in]
    n3220 = Unbundle(w3618) -> ("output high"=w3617:fxp<+/-,64,32>)  [unwired: 1 out]
    n3221 = Divide(x=w3619, y=w3617) -> (x/y=→"Action (%)":dbl)
    n3222 = flat-sequence "To save data" {
      tunnel: [w4988] -> w3926
      tunnel: [w4989] -> w3925
      tunnel: w3879 -> [w4961]
      tunnel: w3659 -> [w4986]
      tunnel: ["Save Calibration"] -> w3900
      tunnel: w3897 -> [w4985]
      tunnel: [w4979] -> w3896
      tunnel: [w4976] -> w3895
      tunnel: [w4973] -> w3894
      tunnel: w3878 -> [w4975]
      tunnel: w3796 -> [w4969]
      tunnel: [w4969] -> w3795
      tunnel: ["Start Saving"] -> w3765
      tunnel: [w4963] -> w3699
      tunnel: [w4962] -> w3698
      tunnel: w3926 -> [w5228]
      tunnel: w3925 -> [w5227]
      tunnel: w3700 -> [w5226]
      tunnel: w3900 -> [w5225]
      tunnel: w3896 -> [w5223]
      tunnel: w3895 -> [w5222]
      tunnel: w3894 -> [w5221]
      tunnel: w3774 -> [w5220]
      tunnel: w3805 -> [w5219]
      tunnel: w3795 -> [w5218]
      tunnel: w3765 -> [w5217]
      tunnel: w3763 -> [w5216]
      tunnel: w3741 -> [w5215]
      tunnel: w3699 -> [w5214]
      tunnel: w3698 -> [w5213]
      tunnel: w3697 -> [w5212]
      tunnel: w3620 -> [w5211]
      frame #0 {
        n3223 = Or(x="Save N Sets", y="Start Saving") -> (x .or. y?=w4970:bool)
        n3224 = To Double Precision Float(number=w4985) -> (double precision float=w4980:dbl)
        n3225 = Build Array(w4970, "Save Calibration", w4961, w4975) -> (w4984:bool[])
        n3226 = Compound Arithmetic op=OR("Save Calibration", w4961, w4970, w4975) -> (w4987:bool)
        n3227 = Boolean Array To Number(Boolean array=w4984) -> (number=w4982:u32)
        n3228 = feedback #32(FALSE ("Save APD Data\nwith Trap Data")) -> (w4964:bool)
        n3229 = feedback #33(refnum<k0> refnum) -> (w4990:refnum<file>)
        n3230 = feedback #34(refnum<k0> refnum) -> (w4966:refnum<file>)
        n3231 = feedback #35(FALSE ("Save APD Data\nwith Trap Data")) -> (w4974:bool)
        n3232 = feedback #36(refnum<k0> refnum) -> (w4977:refnum<file>)
        n3233 = feedback #37(0) -> (w4992:i32)
        n3234 = feedback #38() -> (w4981:u32)  [unwired: 1 out]
        n3235 = case shown="True" w4987 {
          tunnel: [w4999 1] -> w4988
          tunnel: w4992 -> [w5001 _]
          tunnel: [w5000 w5019] -> w4989
          tunnel: w4990 -> [w5000 _]
          tunnel: w4986 -> [_ w5039]
          tunnel: w4980 -> [_ w5037]
          tunnel: w4982 -> [_ w5040]
          tunnel: [w4998 w5018] -> w4979
          tunnel: w4981 -> [w4998 _]
          tunnel: [w4997 w5016] -> w4976
          tunnel: w4977 -> [w4997 _]
          tunnel: [w4996 w5015] -> w4973
          tunnel: w4974 -> [w4996 _]
          tunnel: "Start Saving" -> [_ w5013]
          tunnel: w4969 -> [_ w5012]
          tunnel: [w4995 w5003] -> w4962
          tunnel: w4966 -> [w4995 _]
          tunnel: [w4994 w5002] -> w4963
          tunnel: w4964 -> [w4994 _]
          frame False {
            n3236 = Increment(x=w5001) -> (x+1=w4999:i32)
          }
          frame True {
            w5009 = FALSE ("Start Saving")
            w5014 = 9.0  # File Version
            w5022 = FALSE ("prepend array or string size? (T)")
            w5020 = T29."big-endian, network order" ("byte order (0:big-endian, network order)")
            n3237 = local read "BD 1 Frequency 1 (MHz)"() -> (w5036:dbl)
            n3238 = local read "BD 2 Frequency 1 (MHz)"() -> (w5035:dbl)
            n3239 = local read "BD 1 Frequency 2 (MHz)"() -> (w5034:dbl)
            n3240 = local read "BD 2 Frequency 2 (MHz)"() -> (w5033:dbl)
            n3241 = local read "BD 1 Frequency 3 (MHz)"() -> (w5032:dbl)
            n3242 = local read "BD 2 Frequency 3 (MHz)"() -> (w5031:dbl)
            n3243 = Array Size(array=w5012) -> (size(s)=w5011:i32)
            n3244 = To Double Precision Float(number=w5011) -> (double precision float=w5010:dbl)
            n3245 = local write "Save Calibration"(w5009) -> ()
            n3246 = local write "Start Saving"(w5009) -> ()
            n3247 = Build Array("Save APD Data\nwith Trap Data", "Save Trap Pos. Data") -> (w5006:bool[])
            n3248 = Boolean Array To Number(Boolean array=w5006) -> (number=w5005:u32)
            n3249 = Build Array(w5036, w5035, w5034, w5033, w5032, w5031) -> (w5030:dbl[])
            n3250 = case shown="1, Default" w5040 {
              tunnel: w5039 -> [w5113 w5135 w5151 w5189]
              tunnel: w5010 -> [w5118 w5142 w5171 w5208]
              tunnel: w5037 -> [w5117 w5141 w5170 w5207]
              tunnel: [w5114 w5137 w5162 w5199] -> w5028
              tunnel: [w5106 "Cal sets to save" w5152 w5190] -> w5018
              tunnel: w5030 -> [w5115 w5138 w5164 w5201]
              tunnel: "Save APD Data\nwith Trap Data" -> [w5112 _ w5148 w5187]
              tunnel: [w5112 FALSE ("Save APD Data\nwith Trap Data") w5148 w5187] -> w5015
              tunnel: w5014 -> [w5109 w5132 w5146 w5185]
              tunnel: w5013 -> [w5108 _ _ _]
              tunnel: [w5100 "Active cal?" w5145 w5175] -> w5002
              tunnel: "Save Trap Pos. Data" -> [w5100 _ w5145 w5175]
              tunnel: w5005 -> [w5099 _ w5144 w5174]
              frame 1, Default {
                # "timeseries"
                n3251 = case shown="True" "Profile" {
                  tunnel: [w5121 w5125] -> w5104
                  tunnel: [w5121 w5124] -> w5103
                  tunnel: [w5121 w5123] -> w5102
                  tunnel: [w5121 w5122] -> w5101
                  frame False {
                    w5121 = 0.0 ("f")
                  }
                  frame True {
                    n3252 = local read "Current Position"() -> (w5126:cluster{dbl, dbl, dbl})
                    n3253 = local read "Y change (mm)"() -> (w5122:dbl)
                    n3254 = Unbundle(w5126) -> (w5125:dbl, w5124:dbl, w5123:dbl)
                  }
                }
                n3255 = local read "Save ave N"() -> (w5120:dbl)
                n3256 = Multiply(x=w5120, y=w5113) -> (x*y=w5119:dbl)
                n3257 = To Double Precision Float(number=w5099) -> (double precision float=w5111:dbl)
                n3258 = Select(t=4.0, s="Profile", f=0.0) -> (s? t:f=w5095:dbl)
                n3259 = Build Array(w5109, w5113, w5119, w5118, w5117, w5095) -> (w5116:dbl[])
                n3260 = Build Array(w5111, w5104, w5103, w5102, w5101) -> (w5110:dbl[])
                n3261 = Select(t=u32 4000000000, s=w5108, f="N sets to save") -> (s? t:f=w5106:u32)
                n3262 = Build Array (concatenate)(w5116, w5115, w5110) -> (w5114:dbl[])
              }
              frame 2 {
                w5134 = 0.0 ("f")
                # "If doing active calibration,\nalso save trap position file"
                # "calibration"
                n3263 = property on="Wiggle" class="Bool (strict)"("Val(Sgnl)"="Active cal?") -> ()  [unwired: 2 in, 2 out]
                n3264 = Select(t=2.0, s="Active cal?", f=0.0) -> (s? t:f=w5128:dbl)
                n3265 = Build Array(w5128, w5134, w5134, w5134, w5134) -> (w5133:dbl[])
                n3266 = Build Array(w5132, w5135, w5135, w5142, w5141, 1.0 ("t")) -> (w5139:dbl[])
                n3267 = Build Array (concatenate)(w5139, w5138, w5133) -> (w5137:dbl[])
                "Calibrating..." <- TRUE ("Calibrating...")
              }
              frame 4 {
                w5149 = 0.0 ("f")
                # "scan dir (x/y = 0/1)"
                # "cycles/step"
                # "n scans (f/b)"
                # "steps"
                # "freq. range"
                # "AOD raster scan"
                n3268 = local read "Number of F/B Scans (AOD)"() -> (w5156:u16)
                n3269 = local read "Cycles/step (AOD)"() -> (w5158:u64)
                n3270 = local read "Scan Range (MHz)"() -> (w5161:dbl)
                n3271 = local read "Scan steps (AOD)"() -> (w5160:u64)
                n3272 = local read "Scan BD"() -> (w5168:bool)
                n3273 = local read "Save ave N"() -> (w5173:dbl)
                n3274 = Boolean To (0,1)(Boolean=w5168) -> (0, 1=w5167:i16)
                n3275 = To Double Precision Float(number=w5156) -> (double precision float=w5155:dbl)
                n3276 = To Double Precision Float(number=w5160) -> (double precision float=w5159:dbl)
                n3277 = To Double Precision Float(number=w5158) -> (double precision float=w5157:dbl)
                n3278 = To Double Precision Float(number=w5167) -> (double precision float=w5166:dbl)
                n3279 = Multiply(x=w5173, y=w5151) -> (x*y=w5172:dbl)
                n3280 = To Double Precision Float(number=w5144) -> (double precision float=w5150:dbl)
                n3281 = Build Array(w5150, w5149, w5149, w5149, w5149) -> (w5147:dbl[])
                n3282 = local read "N sets should be saved"() -> (w5153:dbl)
                n3283 = Build Array(w5166, w5161, w5159, w5157, w5155) -> (w5163:dbl[])
                n3284 = Build Array(w5146, w5151, w5172, w5171, w5170, 2.0 ("t")) -> (w5165:dbl[])
                n3285 = Round Toward +Infinity(x=w5153) -> (ceil(x): smallest int >= x=w5154:dbl)
                n3286 = Build Array (concatenate)(w5165, w5164, w5147, w5163) -> (w5162:dbl[])
                n3287 = To Unsigned Long Integer(number=w5154) -> (unsigned 32bit integer=w5152:u32)
              }
              frame 8 {
                w5182 = 0.0 ("f")
                # "MCL raster scan"
                n3288 = local read "Number of scans (MCL)"() -> (w5177:u64)
                n3289 = local read "Scan lines (y)"() -> (w5176:u64)
                n3290 = local read "2D or 1D Scan"() -> (w5179:bool)
                n3291 = local read "Scan Range (V)\n(of steps)"() -> (w5198:dbl)
                n3292 = local read "Fast Scan Dir"() -> (w5205:bool)
                n3293 = local read "Cycles/step (MCL)"() -> (w5195:u64)
                n3294 = local read "Scan steps (MCL)"() -> (w5197:u64)
                n3295 = Select(t=w5176, s=w5179, f=w5177) -> (s? t:f=w5178:u64)
                n3296 = Boolean To (0,1)(Boolean=w5179) -> (0, 1=w5181:i16)
                n3297 = local read "Save ave N"() -> (w5210:dbl)
                n3298 = local read "Initial X"() -> (w5184:dbl)
                n3299 = local read "Initial Y"() -> (w5183:dbl)
                n3300 = To Double Precision Float(number=w5181) -> (double precision float=w5180:dbl)
                n3301 = Boolean To (0,1)(Boolean=w5205) -> (0, 1=w5204:i16)
                n3302 = To Double Precision Float(number=w5178) -> (double precision float=w5193:dbl)
                n3303 = To Double Precision Float(number=w5197) -> (double precision float=w5196:dbl)
                n3304 = To Double Precision Float(number=w5195) -> (double precision float=w5194:dbl)
                n3305 = To Double Precision Float(number=w5204) -> (double precision float=w5203:dbl)
                n3306 = Multiply(x=w5210, y=w5189) -> (x*y=w5209:dbl)
                n3307 = To Double Precision Float(number=w5174) -> (double precision float=w5188:dbl)
